vi "Autonomous Independent.vi"() -> ()   [LabVIEW 2019]
doc: "This VI is called when autonomous begins, and will automatically be terminated when autonomous ends. You can carry out timed or sensor driven robot movement independently without needing to return to the caller."
uses:
  <vilib>/Rock Robotics/Network Tables/NT Read String.vi
  <vilib>/Rock Robotics/WPI/Utilities/WPI_GetSetVariantRefNum.vi
  <vilib>/Rock Robotics/WPI/RobotDrive/WPI_RobotDriveArcadeDrive_Standard(NoSaturation).vi
panel:
  in  "?":i32=127
  in  "Drive Motors Name":string="RobotDrive"
  in  "Speed Value":dbl
  in  "Gyro Name":string="RobotDrive"
  # "Be sure to right-click and choose Data Operations>>Make Current Value default if you want to save the array values with the VI"
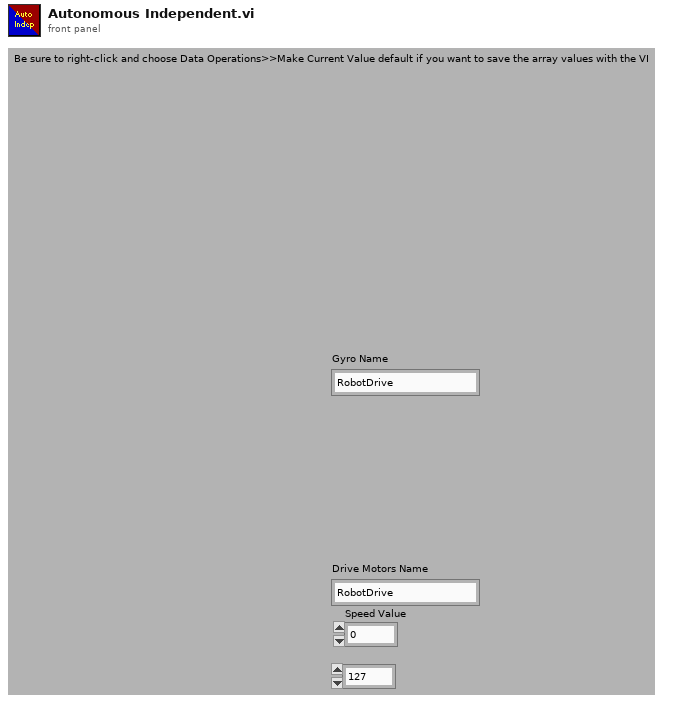
[diagram p1: front panel]
types:
  T1 = typedef "WPI_MotorControlDeviceRef.ctl" = cluster{"DeviceStatus":errorcluster, "Type":T2, "PWM":cluster{"PWM Channel":T3, "DeadBand":T4}, "CAN":cluster{"Device Number":u8, "SetOutput VI Ref":variant, "GetOutput VI Ref":variant, "Enable VI Ref":variant, "Disable VI Ref":variant, "Data":variant}, "Invert":bool, "DIO PWM":cluster{"PWM \"Enable\" Channel":T3, "DIOChannel":T5, "PWM Rate":dbl}}
  T2 = typedef "WPI_MotorControlType.ctl" = enum16{"PWM", "CAN", "DIO PWM"}
  T3 = typedef "FPGA_DIOPWMChannel.ctl" = enum8{"PWM 0", "PWM 1", "PWM 2", "PWM 3", "PWM 4", "PWM 5", "PWM 6", "PWM 7", "PWM 8", "PWM 9", "PWM MXP 0", "PWM MXP 1", "PWM MXP 2", "PWM MXP 3", "PWM MXP 4", "PWM MXP 5", "PWM MXP 6", "PWM MXP 7", "PWM MXP 8", "PWM MXP 9", "Invalid"}
  T4 = typedef "WPI_PWMDeadband.ctl" = cluster{"Name":string, "maxPositivePwm":i32, "minPositivePwm":i32, "centerPwm":i32, "maxNegativePwm":i32, "minNegativePwm":i32, "angularRange":u16}
  T5 = typedef "FPGA_DIOChannel.ctl" = enum8{"DIO 0", "DIO 1", "DIO 2", "DIO 3", "DIO 4", "DIO 5", "DIO 6", "DIO 7", "DIO 8", "DIO 9", "DIO MXP 0", "DIO MXP 1", "DIO MXP 2", "DIO MXP 3", "DIO MXP 4", "DIO MXP 5", "DIO MXP 6", "DIO MXP 7", "DIO MXP 8", "DIO MXP 9", "DIO MXP 10", "DIO MXP 11", "DIO MXP 12", "DIO MXP 13", "DIO MXP 14", "DIO MXP 15", "SPI Port CS1", "SPI Port CS2", "SPI Port CS3", "SPI Port MISO", "SPI Port MOSI", "Invalid"}
  T6 = typedef "WPI_RobotDriveDevRef.ctl" = cluster{"DevStatus":errorcluster, "Motors[]":T1[], "Square Inputs":bool, "Max Output":dbl}
  T7 = typedef "WPI_GyroDevRef.ctl" = cluster{"DevStatus":errorcluster, "Analog Channel":T8, "Gain (VoltsPerDegree/Second)":dbl, "Gyro Type":enum16{"Analog", "XRS450"}, "Handle":i32, "SPI Bus":T9, "Device Found":bool, "Sample Rate":dbl, "Calibrate On Open":bool, "Offset":dbl}
  T8 = typedef "FPGA_AIChannel.ctl" = enum8{"AI 0", "AI 1", "AI 2", "AI 3", "AI MXP 0", "AI MXP 1", "AI MXP 2", "AI MXP 3", "Invalid"}
  T9 = typedef "spi_bus.ctl" = enum16{"SPI On-Board, CS0", "SPI On-Board, CS1", "SPI On-Board, CS2", "SPI On-Board, CS3", "SPI MXP", "Invalid"}
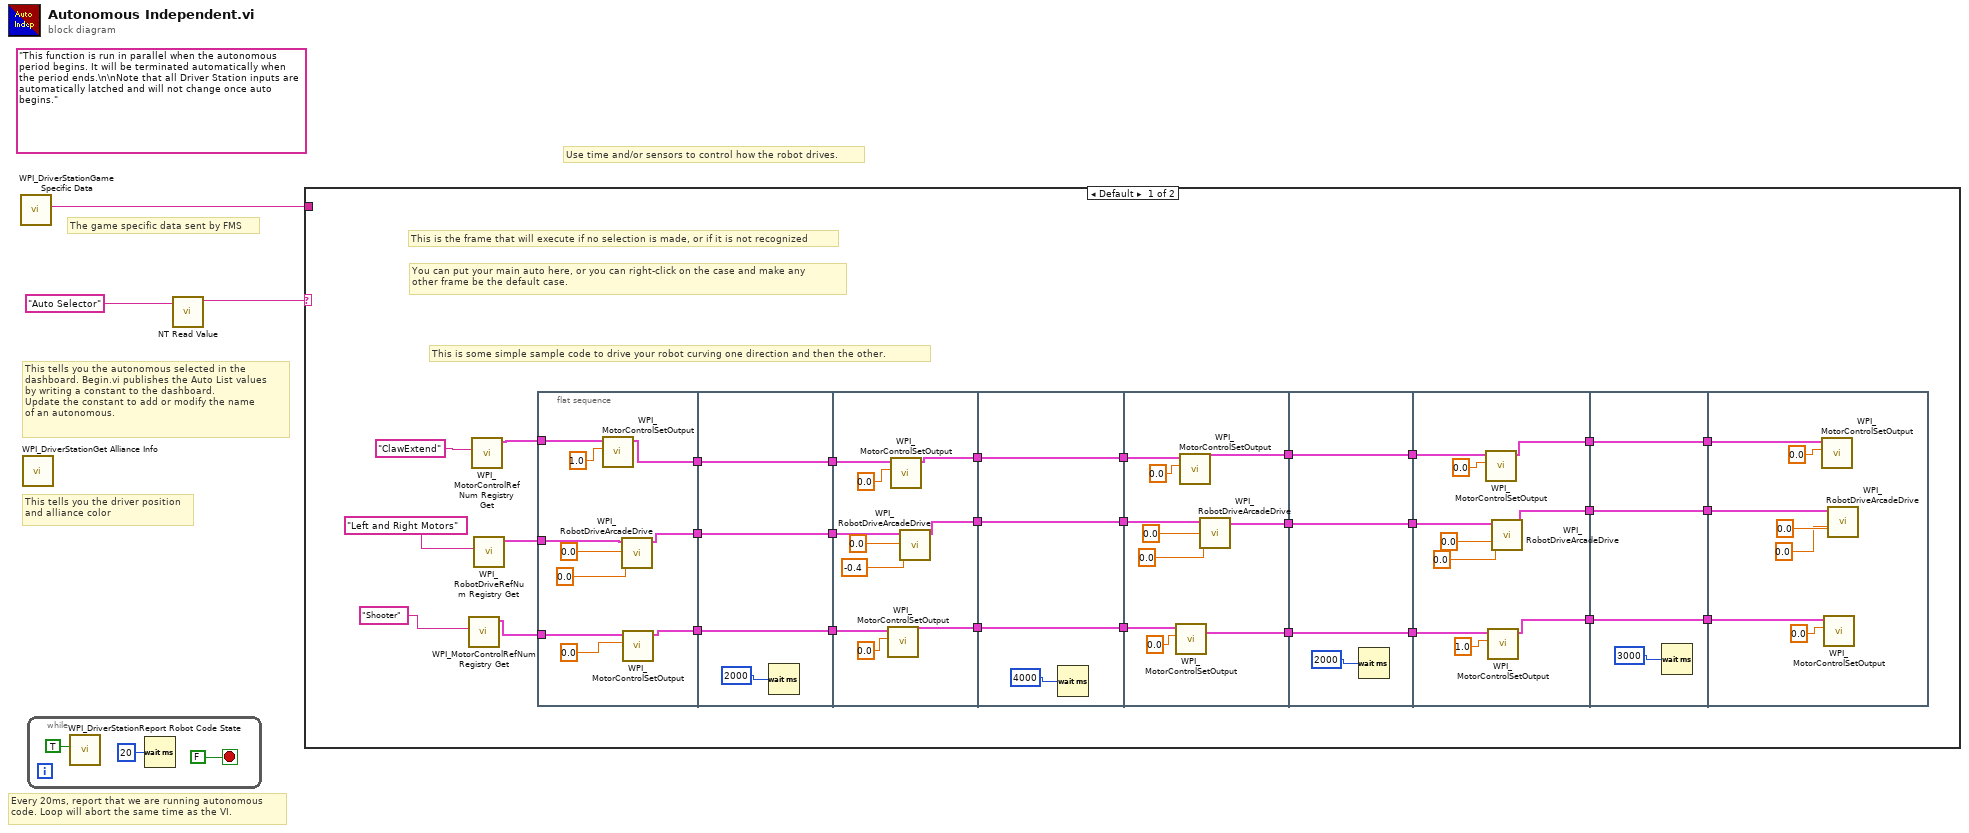
[diagram p0: block diagram]
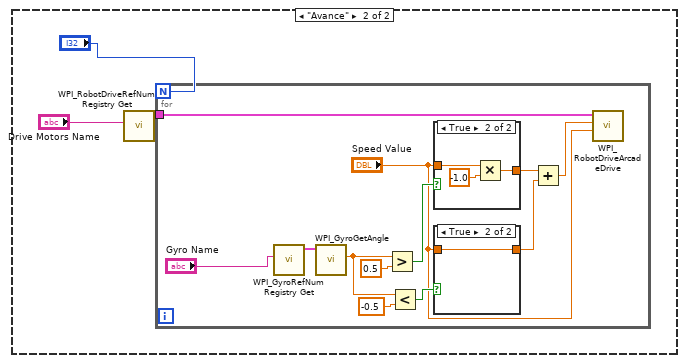
[diagram p2: hidden frame]
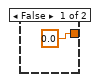
[diagram p3: hidden frame]
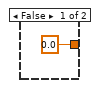
[diagram p4: hidden frame]
diagram:
  (unwired) "This function is run in parallel when the autonomous period begins. It will be terminated automatically when the period ends.\n\nNote that all Driver Station inputs are automatically latched and will not change once auto begins."
  # "The game specific data sent by FMS"
  # "This tells you the autonomous selected in the \ndashboard. Begin.vi publishes the Auto List values\nby writing a constant to the dashboard.\nUpdate the constant to add or modify the name\nof an autonomous."
  # "Every 20ms, report that we are running autonomous\ncode. Loop will abort the same time as the VI."
  # "Use time and/or sensors to control how the robot drives."
  # "This tells you the driver position\nand alliance color"
  n1 = call <vilib>:"WPI_DriverStationGame Specific Data.vi"() -> ("Game Specific Data"=w1:string)  [unwired: 11 in]
  n2 = call <vilib>:"WPI_DriverStationGet Alliance Info.vi"() -> ()  [unwired: 12 out]
  n3 = while {
    stop <- FALSE stop-if-true
    n4 = call <vilib>:"WPI_DriverStationReport Robot Code State.vi"("Autonomous"=TRUE) -> ()  [unwired: 10 in, 1 out]
    n5 = Wait (ms)(milliseconds to wait=u32 20) -> ()  [unwired: 1 out]
  }
  n6 = call-poly <vilib>:"NT Read Value.vi"("Name"="Auto Selector") -> ("String"=w2:string)  [unwired: 9 in, 1 out]
  n7 = case shown="Default" w2 {
    tunnel: w1 -> [_ _]
    frame Default {
      # "This is some simple sample code to drive your robot curving one direction and then the other."
      # "You can put your main auto here, or you can right-click on the case and make any\nother frame be the default case."
      # "This is the frame that will execute if no selection is made, or if it is not recognized"
      n8 = call <vilib>:"WPI_MotorControlRefNum Registry Get.vi"("refnum name"="Shooter") -> ("MotorControlDevRef"=w31:T1)  [unwired: 9 in, 1 out]
      n9 = call <vilib>:"WPI_MotorControlRefNum Registry Get.vi"("refnum name"="ClawExtend") -> ("MotorControlDevRef"=w33:T1)  [unwired: 9 in, 1 out]
      n10 = call <vilib>:"WPI_RobotDriveRefNum Registry Get.vi"("refnum name"="Left and Right Motors") -> ("RobotDriveDevRef"=w32:T6)  [unwired: 9 in, 1 out]
      n11 = flat-sequence {
        tunnel: w33 -> [w46]
        tunnel: w32 -> [w44]
        tunnel: w31 -> [w41]
        tunnel: [w39] -> w30
        tunnel: [w38] -> w28
        tunnel: [w37] -> w26
        tunnel: w30 -> [w49]
        tunnel: [w49] -> w29
        tunnel: w28 -> [w48]
        tunnel: [w48] -> w27
        tunnel: w26 -> [w47]
        tunnel: [w47] -> w25
        tunnel: w29 -> [w59]
        tunnel: w27 -> [w58]
        tunnel: w25 -> [w55]
        tunnel: [w53] -> w24
        tunnel: [w52] -> w22
        tunnel: [w51] -> w20
        tunnel: w24 -> [w63]
        tunnel: [w63] -> w23
        tunnel: w22 -> [w62]
        tunnel: [w62] -> w21
        tunnel: w20 -> [w61]
        tunnel: [w61] -> w19
        tunnel: w23 -> [w74]
        tunnel: w21 -> [w72]
        tunnel: w19 -> [w69]
        tunnel: [w67] -> w18
        tunnel: [w66] -> w16
        tunnel: [w65] -> w14
        tunnel: w18 -> [w77]
        tunnel: [w77] -> w17
        tunnel: w16 -> [w76]
        tunnel: [w76] -> w15
        tunnel: w14 -> [w75]
        tunnel: [w75] -> w13
        tunnel: w17 -> [w88]
        tunnel: w15 -> [w86]
        tunnel: w13 -> [w83]
        tunnel: [w81] -> w12
        tunnel: [w80] -> w10
        tunnel: [w79] -> w8
        tunnel: w12 -> [w92]
        tunnel: [w92] -> w11
        tunnel: w10 -> [w91]
        tunnel: [w91] -> w9
        tunnel: w8 -> [w90]
        tunnel: [w90] -> w7
        tunnel: w11 -> [w96]
        tunnel: w9 -> [w95]
        tunnel: w7 -> [w93]
        frame #0 {
          n12 = call <vilib>:"WPI_MotorControlSetOutput.vi"("Output"=1.0, "MotorControlDevRef"=w46) -> ("MotorControlDevRef"=w39:T1)  [unwired: 7 in, 2 out]
          n13 = call-poly <vilib>:"WPI_RobotDriveArcadeDrive.vi"("Y axis value"=0.0, "X axis value"=0.0, "RobotDriveDevRef"=w44) -> ("RobotDriveDevRef"=w38:T6)  [unwired: 6 in, 2 out]
          n14 = call <vilib>:"WPI_MotorControlSetOutput.vi"("Output"=0.0, "MotorControlDevRef"=w41) -> ("MotorControlDevRef"=w37:T1)  [unwired: 7 in, 2 out]
        }
        frame #1 {
          n15 = Wait (ms)(milliseconds to wait=u32 2000) -> ()  [unwired: 1 out]
        }
        frame #2 {
          n16 = call <vilib>:"WPI_MotorControlSetOutput.vi"("Output"=0.0, "MotorControlDevRef"=w55) -> ("MotorControlDevRef"=w51:T1)  [unwired: 7 in, 2 out]
          n17 = call <vilib>:"WPI_MotorControlSetOutput.vi"("Output"=0.0, "MotorControlDevRef"=w59) -> ("MotorControlDevRef"=w53:T1)  [unwired: 7 in, 2 out]
          n18 = call-poly <vilib>:"WPI_RobotDriveArcadeDrive.vi"("Y axis value"=-0.4, "X axis value"=0.0, "RobotDriveDevRef"=w58) -> ("RobotDriveDevRef"=w52:T6)  [unwired: 6 in, 2 out]
        }
        frame #3 {
          n19 = Wait (ms)(milliseconds to wait=u32 4000) -> ()  [unwired: 1 out]
        }
        frame #4 {
          n20 = call <vilib>:"WPI_MotorControlSetOutput.vi"("Output"=0.0, "MotorControlDevRef"=w69) -> ("MotorControlDevRef"=w65:T1)  [unwired: 7 in, 2 out]
          n21 = call <vilib>:"WPI_MotorControlSetOutput.vi"("Output"=0.0, "MotorControlDevRef"=w74) -> ("MotorControlDevRef"=w67:T1)  [unwired: 7 in, 2 out]
          n22 = call-poly <vilib>:"WPI_RobotDriveArcadeDrive.vi"("Y axis value"=0.0, "X axis value"=0.0, "RobotDriveDevRef"=w72) -> ("RobotDriveDevRef"=w66:T6)  [unwired: 6 in, 2 out]
        }
        frame #5 {
          n23 = Wait (ms)(milliseconds to wait=u32 2000) -> ()  [unwired: 1 out]
        }
        frame #6 {
          n24 = call <vilib>:"WPI_MotorControlSetOutput.vi"("Output"=0.0, "MotorControlDevRef"=w88) -> ("MotorControlDevRef"=w81:T1)  [unwired: 7 in, 2 out]
          n25 = call <vilib>:"WPI_MotorControlSetOutput.vi"("Output"=1.0, "MotorControlDevRef"=w83) -> ("MotorControlDevRef"=w79:T1)  [unwired: 7 in, 2 out]
          n26 = call-poly <vilib>:"WPI_RobotDriveArcadeDrive.vi"("Y axis value"=0.0, "X axis value"=0.0, "RobotDriveDevRef"=w86) -> ("RobotDriveDevRef"=w80:T6)  [unwired: 6 in, 2 out]
        }
        frame #7 {
          n27 = Wait (ms)(milliseconds to wait=u32 3000) -> ()  [unwired: 1 out]
        }
        frame #8 {
          n28 = call <vilib>:"WPI_MotorControlSetOutput.vi"("Output"=0.0, "MotorControlDevRef"=w96) -> ()  [unwired: 7 in, 3 out]
          n29 = call <vilib>:"WPI_MotorControlSetOutput.vi"("Output"=0.0, "MotorControlDevRef"=w93) -> ()  [unwired: 7 in, 3 out]
          n30 = call-poly <vilib>:"WPI_RobotDriveArcadeDrive.vi"("Y axis value"=0.0, "X axis value"=0.0, "RobotDriveDevRef"=w95) -> ()  [unwired: 6 in, 3 out]
        }
      }
    }
    frame "Avance" {
      n31 = call <vilib>:"WPI_RobotDriveRefNum Registry Get.vi"("refnum name"="Drive Motors Name") -> ("RobotDriveDevRef"=w102:T6)  [unwired: 9 in, 1 out]
      n32 = for {
        N: "?" -> [_]
        tunnel: w102 -> [w114]
        n33 = call <vilib>:"WPI_GyroRefNum Registry Get.vi"("refnum name"="Gyro Name") -> ("GyroDevRef"=w113:T7)  [unwired: 9 in, 1 out]
        n34 = call <vilib>:"WPI_GyroGetAngle.vi"("GyroDevRef"=w113) -> ("Angle"=w111:dbl)  [unwired: 6 in, 4 out]
        n35 = Greater?(x=w111, y=0.5) -> (0:w108:bool)
        n36 = Less?(x=w111, y=-0.5) -> (x < y?=w112:bool)
        n37 = case shown="True" w108 {
          tunnel: [0.0 w120] -> w106
          tunnel: "Speed Value" -> [_ w118]
          frame False {
          }
          frame True {
            n38 = Multiply(x=w118, y=-1.0) -> (x*y=w120:dbl)
          }
        }
        n39 = case shown="True" w112 {
          tunnel: [0.0 w116] -> w107
          tunnel: "Speed Value" -> [_ w116]
          frame False {
          }
          frame True {
          }
        }
        n40 = Add(x=w106, y=w107) -> (x+y=w105:dbl)
        n41 = call-poly <vilib>:"WPI_RobotDriveArcadeDrive.vi"("Y axis value"="Speed Value", "X axis value"=w105, "RobotDriveDevRef"=w114) -> ()  [unwired: 6 in, 3 out]
      }
    }
  }
